vi "PAN_ToLog.vi"(9 "message":string, 10 "type":u16(ring) items=["command", "imediateReply", "CallbackReply", "Information", "AsyncMsg"]) -> ()   [LabVIEW 2016]
panel:
  in  "Message":cluster{"string":string, "type":u16} {"type" items=["command", "imediateReply", "CallbackReply", "Information", "AsyncMsg"]}
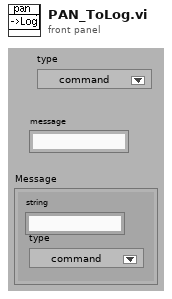
[diagram p1: front panel]
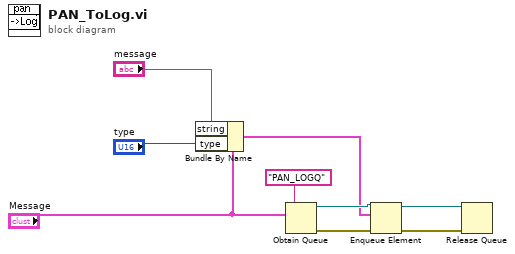
[diagram p0: block diagram]
diagram:
  n1 = Bundle By Name(cluster="Message", "string"="message", "type"="type") -> (w1:cluster{"string":string, "type":u16})
  n2 = Obtain Queue(name (unnamed)="PAN_LOGQ", element data type="Message") -> (queue out=w8:refnum<queue>, error out=w9:errorcluster)  [unwired: 3 in, 1 out]
  n3 = Enqueue Element(queue=w8, element=w1, error in (no error)=w9) -> (queue out=w7:refnum<queue>, error out=w6:errorcluster)  [unwired: 2 out]
  n4 = Release Queue(queue=w7, error in (no error)=w6) -> ()  [unwired: 4 out]
